vi "Read.vi"(8 "error in (no error)":errorcluster, 9 "Variant":variant, 11 "AK TCP in":refnum<class "AK TCP.lvclass">) -> (0 "error out":errorcluster, 2 "String":string, 3 "AK TCP out":refnum<class "AK TCP.lvclass">)   [LabVIEW 2013, in "Protocol Classes.lvlib" / "AK TCP.lvclass"]
uses:
  AK TCP.lvclass
  TCP/TCP.lvclass
  Protocol Parent/Methods/Read Parameter.ctl
  AK TCP.lvclass/AK TCP.ctl
  Data Access/Read Current Command Code.vi
  <vilib>/Utility/error.llb/Error Cluster From Error Code.vi
  Protocol Classes.lvlib
  Protocol Parent/Protocol Parent.lvclass
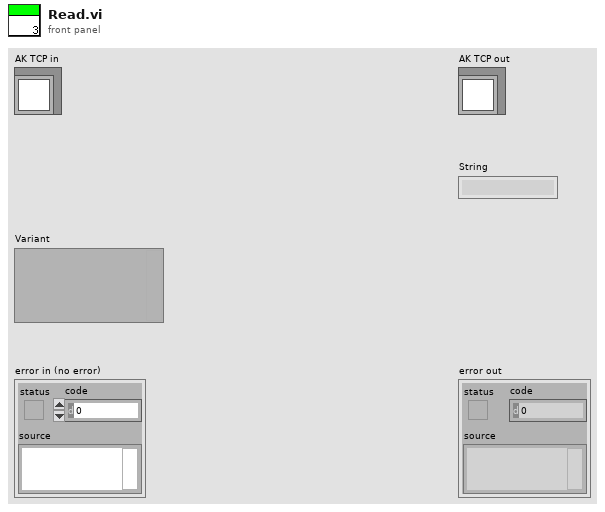
[diagram p1: front panel]
types:
  T1 = typedef "Protocol Classes.lvlib/Protocol Parent.lvclass/Read Parameter.ctl" = cluster{"Wait Type":enum16{"Byte Count", "Wait sec"}, "Wait Value":dbl}
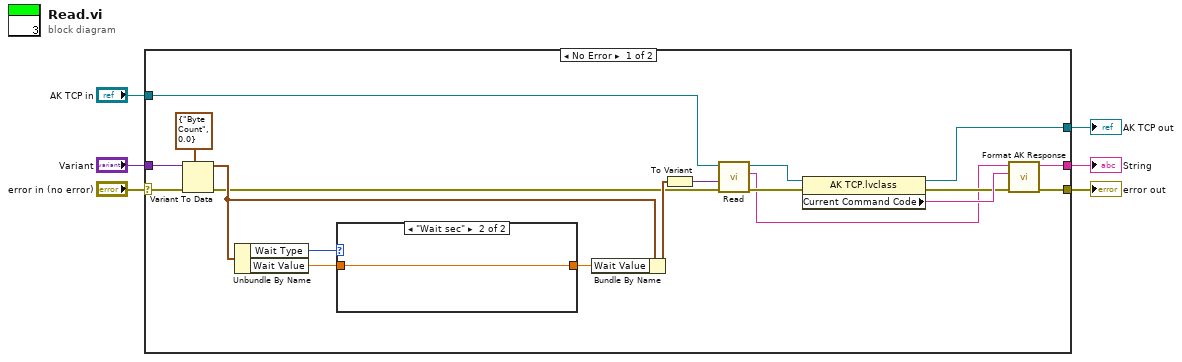
[diagram p0: block diagram]
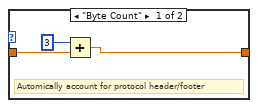
[diagram p2: hidden frame]
diagram:
  n1 = case shown="No Error" "error in (no error)" {
    selector: "error in (no error)" -> [w10 w31]
    tunnel: "Variant" -> [w8 _]
    tunnel: "AK TCP in" -> [w25 w30]
    tunnel: [w22 w30] -> w4
    tunnel: [w20 _] -> w3
    tunnel: [w18 w31] -> w5
    frame No Error {
      n2 = Variant To Data(error in=w10, type=T1 {"Wait Type"=enum."Byte Count", "Wait Value"=0.0} ("Read Parameter"), Variant=w8) -> (data=w14:T1, error out=w9:errorcluster)
      n3 = Unbundle By Name(w14) -> ("Wait Type"=w12:enum16{"Byte Count", "Wait sec"}, "Wait Value"=w13:dbl)
      n4 = case shown="\"Wait sec\"" w12 {
        tunnel: w13 -> [w28 w29]
        tunnel: [w26 w29] -> w15
        frame "Byte Count" {
          # "Automically account for protocol header/footer"
          n5 = Add(x=3, y=w28) -> (x+y=w26:dbl)
        }
        frame "Wait sec" {
        }
      }
      n6 = Bundle By Name(cluster=w14, "Wait Value"=w15) -> (w16:T1)
      n7 = To Variant(anything=w16) -> (Variant=w7:variant)
      n8 = call-parent "Read.vi"("error in (no error)"=w9, "Variant"=w7, "Ethernet in"=w25) -> ("error out"=w24:errorcluster, "String"=w17:string, "Ethernet out"=w23:refnum<class "AK TCP.lvclass">)  [unwired: 6 in]
      n9 = property class="AK TCP.lvclass"(reference=w23, error in=w24) -> (reference out=w22:refnum<class "AK TCP.lvclass">, error out=w19:errorcluster, "Current Command Code"=w21:string)
      n10 = call "Format AK Response.vi"("error in (no error)"=w19, "Current Command Code"=w21, "Response"=w17) -> ("error out"=w18:errorcluster, "Data"=w20:string)  [unwired: 7 in]
    }
    frame Error {
    }
  }
  "error out" <- w5
  "AK TCP out" <- w4
  "String" <- w3
